vi "OpenHelp.vi"(8 "Caller VI":refnum<vi>, 9 "Microprocessor in":T1, 11 "Name":path) -> ()   [LabVIEW 2016, in "uPythonX.xctl"]
uses:
  uPythonX.xctl
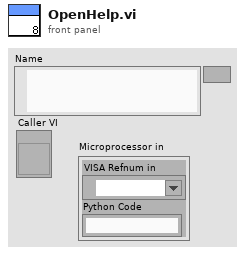
[diagram p1: front panel]
types:
  T1 = cluster{"VISA Refnum in":refnum<visa-resource-name>, "Python Code":string}
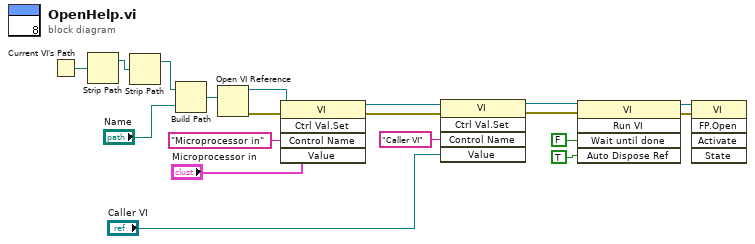
[diagram p0: block diagram]
diagram:
  n1 = Current VI's Path() -> (path=w14:path)
  n2 = Strip Path(path=w14) -> (stripped path=w15:path)  [unwired: 1 out]
  n3 = Strip Path(path=w15) -> (stripped path=w16:path)  [unwired: 1 out]
  n4 = Build Path(base path=w16, name or relative path="Name") -> (appended path=w17:path)
  n5 = Open VI Reference(vi path=w17) -> (vi reference=w8:refnum<vi>, error out=w7:errorcluster)  [unwired: 5 in]
  n6 = invoke class="VI" method="Ctrl Val.Set"(reference=w8, error in=w7, "Control Name"="Microprocessor in", "Value"="Microprocessor in") -> (reference out=w6:refnum<vi>, error out=w5:errorcluster)  [unwired: 1 in, 3 out]
  n7 = invoke class="VI" method="Ctrl Val.Set"(reference=w6, error in=w5, "Control Name"="Caller VI", "Value"="Caller VI") -> (reference out=w4:refnum<vi>, error out=w3:errorcluster)  [unwired: 1 in, 3 out]
  n8 = invoke class="VI" method="Run VI"(reference=w4, error in=w3, "Wait until done"=FALSE ("Wait Until Done"), "Auto Dispose Ref"=TRUE ("Auto Dispose Reference")) -> (reference out=w18:refnum<vi>, error out=w19:errorcluster)  [unwired: 1 in, 3 out]
  n9 = invoke class="VI" method="FP.Open"(reference=w18, error in=w19) -> ()  [unwired: 3 in, 5 out]
